vi "Set AM Properties.vi"(0 "VISA resource name":refnum<visa-resource-name>, 5 "Channel (0: Channel 1)":T1 items=["Channel 1", "Channel 2"], 7 "AM Source (0: Internal)":u16(ring) items=["Internal", "External"], 9 "Modulation Waveform (0: Sine)":u16(ring) items=["Sine", "Square", "Triangle", "Ramp", "Down Ramp", "Noise"], 11 "error in (no error)":errorcluster, 12 "Modulation Frequency (1000 Hz)":dbl[unit]=1000.0, 13 "Modulation Depth (0 %)":dbl) -> (4 "VISA resource name out":refnum<visa-resource-name>, 15 "error out":errorcluster)   [LabVIEW 2017, in "Tektronix AFG 3000 Series.lvlib"]
uses:
  Tektronix AFG 3000 Series.lvlib
  controls.llb/Channel.ctl
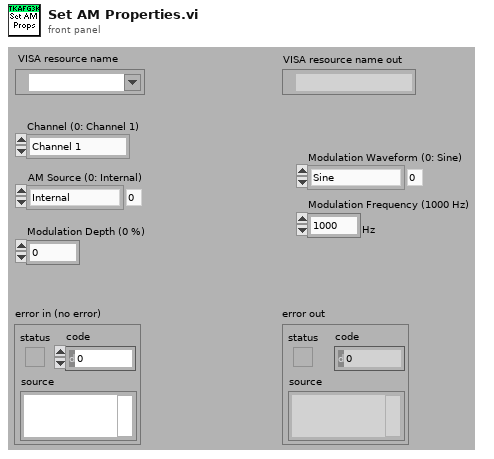
[diagram p1: front panel]
types:
  T1 = typedef "Channel.ctl" = u16
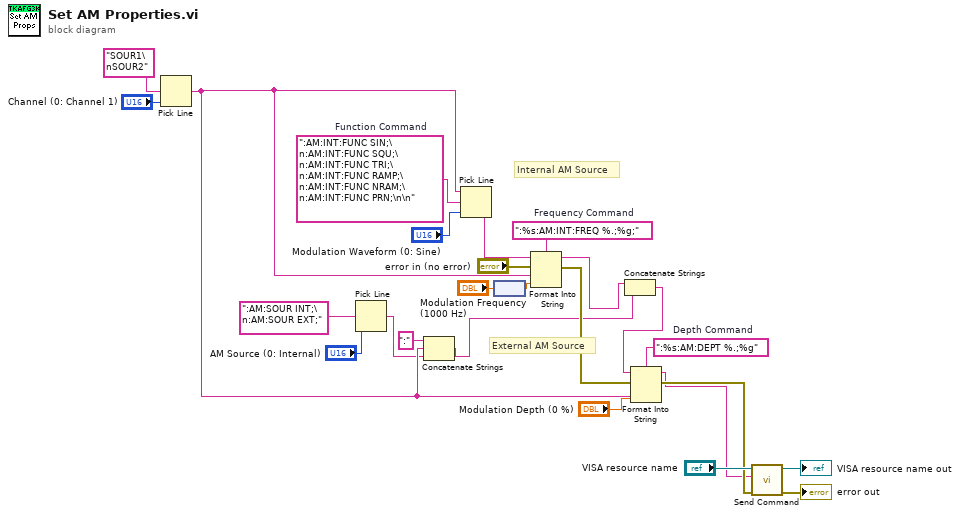
[diagram p0: block diagram]
diagram:
  w18 = ":%s:AM:INT:FREQ %.;%g;"  # Frequency Command
  w19 = ":AM:INT:FUNC SIN;\n:AM:INT:FUNC SQU;\n:AM:INT:FUNC TRI;\n:AM:INT:FUNC RAMP;\n:AM:INT:FUNC NRAM;\n:AM:INT:FUNC PRN;\n\n"  # Function Command
  w22 = ":%s:AM:DEPT %.;%g"  # Depth Command
  # "External AM Source"
  # "Internal AM Source"
  n1 = Pick Line(multi-line string="SOUR1\nSOUR2" ("string (\"\")"), line index="Channel (0: Channel 1)") -> (output string=w3:string)  [unwired: 1 out]
  n2 = Pick Line(multi-line string=":AM:SOUR INT;\n:AM:SOUR EXT;" ("Source Command"), line index="AM Source (0: Internal)") -> (output string=w2:string)  [unwired: 1 out]
  n3 = Concatenate Strings(":" ("string"), w3, w2) -> (w1:string)
  n4 = Pick Line(string ("")=w3, multi-line string=w19, line index="Modulation Waveform (0: Sine)") -> (output string=w17:string)
  n5 = node("Modulation Frequency (1000 Hz)") -> (w12:dbl)
  n6 = Format Into String(format string=w18, initial string=w17, error in="error in (no error)", w3, w12) -> (resulting string=w5:string, error out=w14:errorcluster)
  n7 = Concatenate Strings(w5, w1) -> (w6:string)
  n8 = Format Into String(format string=w22, initial string=w6, error in=w14, w3, "Modulation Depth (0 %)") -> (resulting string=w7:string, error out=w8:errorcluster)
  n9 = call "Send Command.vi"("error in (no error)"=w8, "write buffer"=w7, "VISA resource name"="VISA resource name") -> ("error out"=→"error out":errorcluster, "VISA resource name out"=→"VISA resource name out":refnum<visa-resource-name>)  [unwired: 7 out]
